vi "Set Intensity Scales (Start and End).vi"(7 "Intensity Data":dbl[][](array[numeric]), 8 "error in (no error)":errorcluster, 9 "y start & end":cluster{"y start":dbl, "y end":dbl}, 10 "x start & end":cluster{"x start":dbl, "x end":dbl}, 11 "graph_utilities in":refnum<class "graph_utilities.lvclass">) -> (0 "error out":errorcluster, 3 "graph_utilities out":refnum<class "graph_utilities.lvclass">)   [LabVIEW 2016]
uses:
  <vilib>/Utility/miscctls.llb/LVOffsetAndMultiplierTypeDef.ctl
  graph_utilities.lvclass
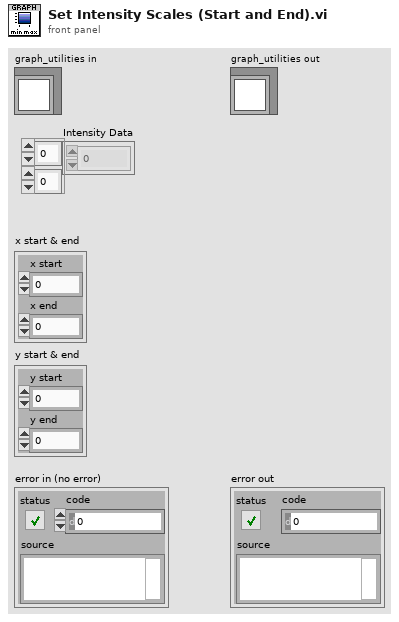
[diagram p1: front panel]
types:
  T1 = typedef "LVOffsetAndMultiplierTypeDef.ctl" = cluster{"Offset":dbl, "Multiplier":dbl}
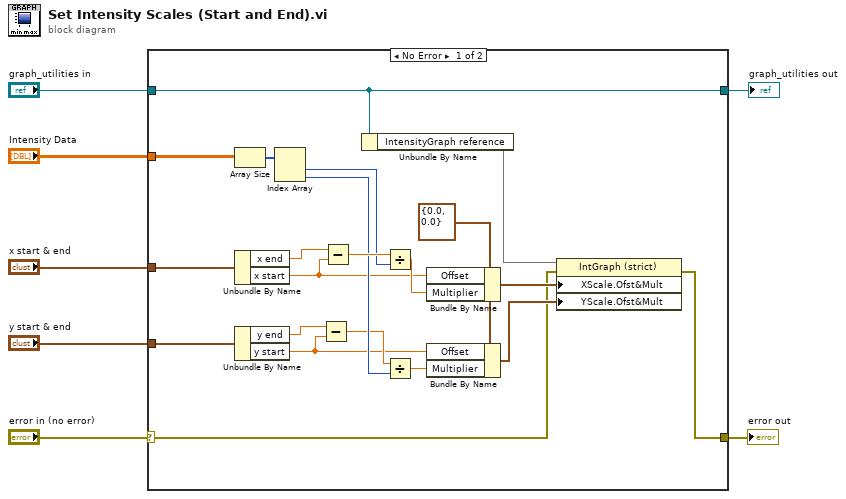
[diagram p0: block diagram]
diagram:
  n1 = case shown="No Error" "error in (no error)" {
    selector: "error in (no error)" -> [w15 w30]
    tunnel: "Intensity Data" -> [w24 _]
    tunnel: "x start & end" -> [w23 _]
    tunnel: "y start & end" -> [w21 _]
    tunnel: [w16 w30] -> w4
    tunnel: "graph_utilities in" -> [w8 w29]
    tunnel: [w8 w29] -> w1
    frame No Error {
      w17 = T1 {"Offset"=0.0, "Multiplier"=0.0} ("X Scale.Offset and Multiplier")
      n2 = Array Size(array=w24) -> (size(s)=w25:i32[])
      n3 = Unbundle By Name(w23) -> ("x end"=w22:dbl, "x start"=w12:dbl)
      n4 = Unbundle By Name(w21) -> ("y end"=w20:dbl, "y start"=w10:dbl)
      n5 = Index Array(array=w25) -> (element #1=w13:i32, element #2=w19:i32)  [unwired: 2 in]
      n6 = Subtract(x=w20, y=w10) -> (x-y=w11:dbl)
      n7 = Subtract(x=w22, y=w12) -> (x-y=w26:dbl)
      n8 = Unbundle By Name(w8) -> ("IntensityGraph reference"=w9)
      n9 = Divide(x=w26, y=w13) -> (x/y=w14:dbl)
      n10 = Divide(x=w11, y=w19) -> (x/y=w27:dbl)
      n11 = Bundle By Name(cluster=w17, "Offset"=w12, "Multiplier"=w14) -> (w28:T1)
      n12 = Bundle By Name(cluster=w17, "Offset"=w10, "Multiplier"=w27) -> (w18:T1)
      n13 = property on="Property Node" class="IntGraph (strict)"(reference=w9, error in=w15, "XScale.Ofst&Mult"=w28, "YScale.Ofst&Mult"=w18) -> (error out=w16:errorcluster)  [unwired: 1 out]
    }
    frame Error {
    }
  }
  "error out" <- w4
  "graph_utilities out" <- w1
